vi "Connection Handler.vi"(6 "connection reference":refnum<data-value>, 8 "UUID":string, 9 "data model":refnum<class "Device Data Model.lvclass">, 10 "transmission data unit":refnum<class "Transmission Data Unit.lvclass">, 11 "TCP slave":refnum<class "TCP Slave.lvclass">) -> ()   [LabVIEW 2020, in "SubVIs.lvlib" / "TCP Slave.lvclass"]
doc: "Handles new connections by waiting on TCP requests. When data is received, it will execute the modbus data unit and write the return data back onto the bus. It handles one request at a time."
uses:
  <vilib>/Modbus/subvis/Protocol/TCP/TCP Slave/TCP Slave.lvclass
  <vilib>/Modbus/subvis/Transmission Data Unit (ADU)/Transmission Data Unit/Transmission Data Unit.lvclass
  C:/builds/penguin/iak/lvdsc/trunk/20.0/lv/vi.lib/Modbus/subvis/Protocol/Interfaces/Network Protocol/Network Protocol.lvclass
  <vilib>/Modbus/subvis/Data and Functions/Device Data Model/Device Data Model.lvclass
  <vilib>/Modbus/subvis/Protocol/TCP/TCP Slave/TCP Slave.lvclass/TCP Slave.ctl
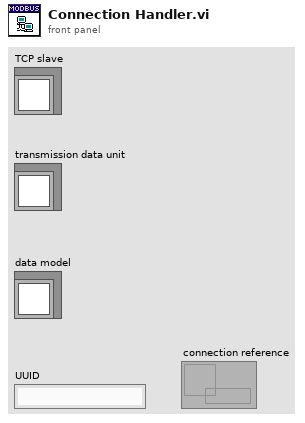
[diagram p1: front panel]
types:
  T1 = enum16{"Check Notifier", "Wait on Connection", "Quit"}
  T2 = cluster{"Connected?":bool, "IP address":string, "connection error":errorcluster}
  T3 = typedef "SubVIs.lvlib/TCP Slave.lvclass/Connection Counter.ctl" = cluster{"Currently Connected":u32, "Connection Records":refnum<data-value>[]}
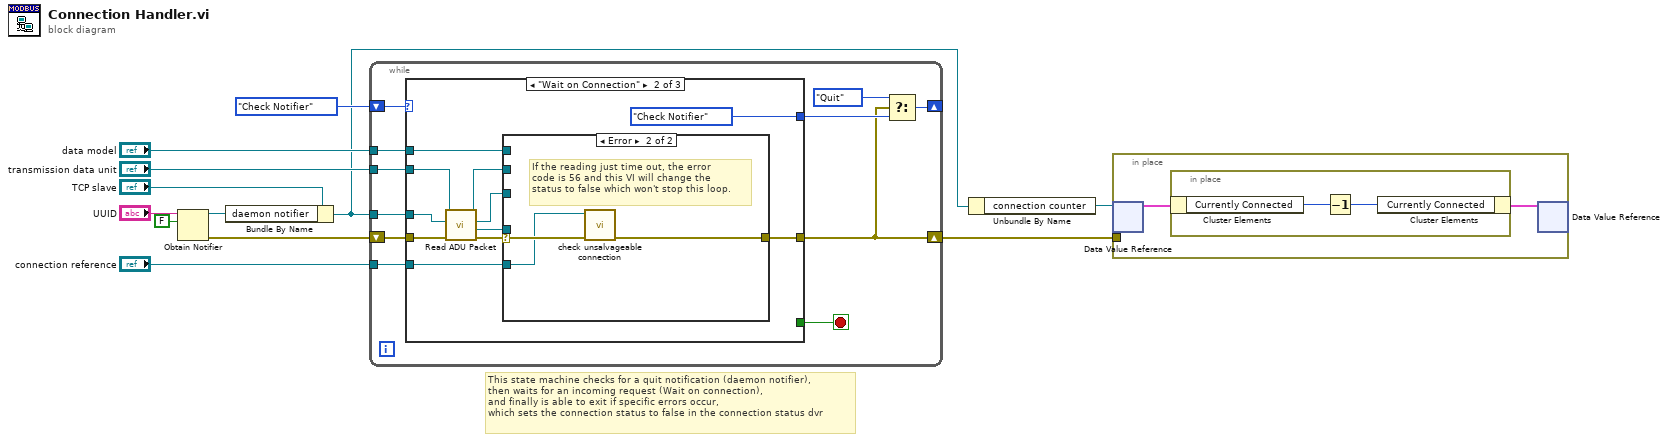
[diagram p0: block diagram]
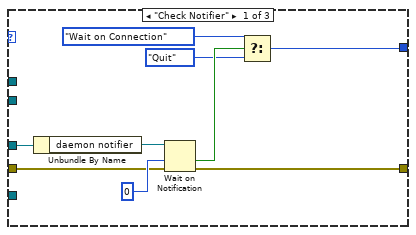
[diagram p2: hidden frame]
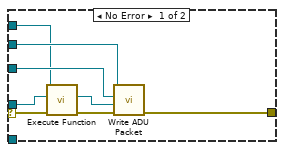
[diagram p3: hidden frame]
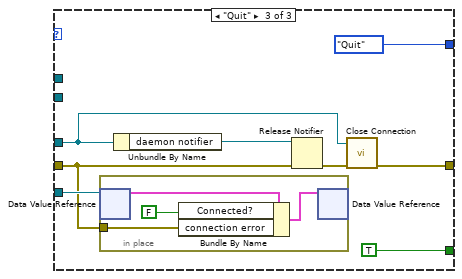
[diagram p4: hidden frame]
diagram:
  # "This state machine checks for a quit notification (daemon notifier),\nthen waits for an incoming request (Wait on connection),\nand finally is able to exit if specific errors occur,\nwhich sets the connection status to false in the connection status dvr"
  n1 = Obtain Notifier(name (unnamed)="UUID", notification data type=FALSE) -> (notifier out=w7:refnum<notifier>, error out=w9:errorcluster)  [unwired: 2 in, 1 out]
  n2 = Bundle By Name(cluster="TCP slave", "daemon notifier"=w7) -> (w1:refnum<class "TCP Slave.lvclass">)
  n3 = while {
    shift-right: [w21] -> _
    shift-left: T1."Check Notifier" ("Listener State") -> [w23]
    shift-right: [w18] -> w3
    shift-left: w9 -> [w17]
    tunnel: w1 -> [w16]
    tunnel: "connection reference" -> [w15]
    tunnel: "transmission data unit" -> [w14]
    tunnel: "data model" -> [w13]
    stop <- w19 stop-if-true
    n4 = case shown="\"Wait on Connection\"" w23 {
      tunnel: [w25 T1."Check Notifier" ("Listener State") T1."Quit" ("Listener State")] -> w20
      tunnel: [_ _ TRUE] -> w19
      tunnel: [w30 w37 w58] -> w18
      tunnel: w17 -> [w29 w38 w55]
      tunnel: w16 -> [w24 w36 w57]
      tunnel: w15 -> [_ w34 w56]
      tunnel: w14 -> [_ w35 _]
      tunnel: w13 -> [_ w33 _]
      frame "Check Notifier" {
        n5 = Unbundle By Name(w24) -> ("daemon notifier"=w31:refnum<notifier>)
        n6 = Wait on Notification(notifier=w31, timeout in ms (-1)=0, error in (no error)=w29) -> (timed out?=w28:bool, error out=w30:errorcluster)  [unwired: 1 in, 2 out]
        n7 = Select(t=T1."Wait on Connection" ("Listener State"), s=w28, f=T1."Quit" ("Listener State")) -> (s? t:f=w25:T1)
      }
      frame "Wait on Connection" {
        n8 = call-dynamic "Read ADU Packet.vi"("error in (no error)"=w38, "protocol layer"=w36, "transmission data unit in"=w35) -> ("error out"=w42:errorcluster, "Modbus data unit"=w40:refnum<class "Modbus Data Unit (PDU).lvclass">, "protocol layer out"=w39:refnum<class "Network Protocol.lvclass">, "transmission data unit out"=w41:refnum<class "Transmission Data Unit.lvclass">)  [unwired: 4 in, 1 out]
        n9 = case shown="Error" w42 {
          selector: w42 -> [w46 w54]
          tunnel: w41 -> [w51 _]
          tunnel: w40 -> [w50 _]
          tunnel: w39 -> [w48 _]
          tunnel: [w47 w53] -> w37
          tunnel: w34 -> [_ w52]
          tunnel: w33 -> [w44 _]
          frame No Error {
            n10 = call-dynamic "Execute Function.vi"("error in (no error)"=w46, "Modbus request"=w50, "device data model in"=w44) -> ("error out"=w45:errorcluster, "Modbus response"=w49:refnum<class "Modbus Data Unit (PDU).lvclass">)  [unwired: 6 in, 1 out]
            n11 = call-dynamic "Write ADU Packet.vi"("error in (no error)"=w45, "Modbus data unit"=w49, "protocol layer"=w48, "transmission data unit in"=w51) -> ("error out"=w47:errorcluster)  [unwired: 5 in, 2 out]
          }
          frame Error {
            # "If the reading just time out, the error\ncode is 56 and this VI will change the\nstatus to false which won't stop this loop."
            n12 = call <vilib>:"check unsalvageable connection.vi"("error in (no error)"=w54, "connection reference"=w52) -> ("error out"=w53:errorcluster)  [unwired: 9 in]
          }
        }
      }
      frame "Quit" {
        n13 = in-place {
          in-place-border: w55 -> [w63]
          n14 = in-place-dvr #1(w56) -> (w66:T2)  [unwired: 1 out]
          n15 = Bundle By Name(cluster=w66, "Connected?"=FALSE, "connection error"=w63) -> (w64:T2)
          n16 = in-place-dvr #1(w64) -> ()  [unwired: 2 out]
        }
        n17 = Unbundle By Name(w57) -> ("daemon notifier"=w60:refnum<notifier>)
        n18 = Release Notifier(notifier=w60, error in (no error)=w55) -> (error out=w59:errorcluster)  [unwired: 1 in, 2 out]
        n19 = call <vilib>:"Close Connection.vi"("error in (no error)"=w59, "TCP slave in"=w57) -> ("error out"=w58:errorcluster)  [unwired: 9 in]
      }
    }
    n20 = Select(t=T1."Quit" ("Listener State"), s=w18, f=w20) -> (s? t:f=w21:T1)
  }
  n21 = Unbundle By Name(w1) -> ("connection counter"=w2:refnum<data-value>)
  n22 = in-place {
    in-place-border: w3 -> [_]
    n23 = in-place-dvr #2(w2) -> (w68:T3)  [unwired: 1 out]
    n24 = in-place {
      n25 = in-place-cluster #3(w68) -> ("Currently Connected"=w70:u32)
      n26 = Decrement(x=w70) -> (x-1=w69:u32)
      n27 = in-place-cluster #3("Currently Connected"=w69) -> (w67:T3)
    }
    n28 = in-place-dvr #2(w67) -> ()  [unwired: 2 out]
  }
